vi "Rebuild Addon Settings.vi"(8 "error in (no error)":errorcluster, 11 "Section Ref in":T1 format="%.0x") -> (0 "error out":errorcluster, 3 "Parent Ref out":T1 format="%.0x")   [LabVIEW 2013, in "J1939 Addon System Explorer.lvlib"]
uses:
  J1939 Addon System Explorer.lvlib
  <vilib>/NI Veristand/Custom Device API/Custom Device Item Ref.ctl
  Shared/SubVIs/Constants.vi
  <vilib>/NI Veristand/Custom Device Tools/Custom Device Utility Library/NI VeriStand - Search for Item by Name.vi
  <vilib>/NI Veristand/Custom Device API/Custom Device API.lvlib
  Shared/J1939 Addon Shared.lvlib
  <vilib>/NI Veristand/Custom Device Tools/Custom Device Utility Library/Custom Device Utility Library.lvlib
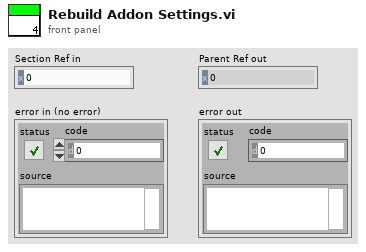
[diagram p1: front panel]
types:
  T1 = typedef "Custom Device API.lvlib/Custom Device Item Ref.ctl" = u64
  T2 = typedef "J1939 Addon Shared.lvlib/XNET Frame Event Properties.ctl" = cluster{"Transmit trigger":enum16{"Channel value change"}, "Enable software cyclic trigger":bool, "Transmit Time":dbl}
  T3 = typedef "J1939 Addon Shared.lvlib/SPN Properties.ctl" = cluster{"Bytes":u32, "ScaleFac":dbl, "ScaleOff":dbl}
  T4 = cluster{"Name":string, "ID":u32, "Frame Transmit Info":T2, "Signal List":cluster{"Name":string, "SPN":T3}[]}[]
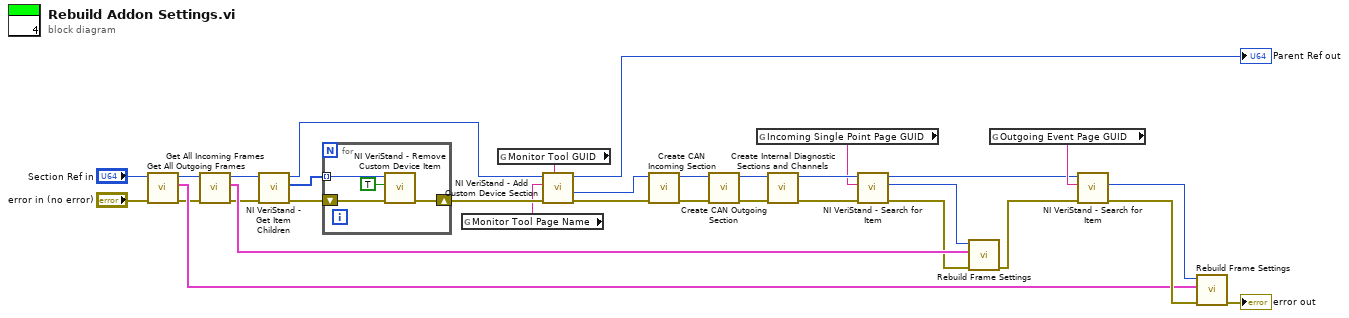
[diagram p0: block diagram]
diagram:
  n1 = call "Get All Outgoing Frames.vi"("error in"="error in (no error)", "Item Ref"="Section Ref in") -> ("error out"=w3:errorcluster, "Frames"=w7:T4, "Item Ref out"=w4:T1)  [unwired: 7 in]
  n2 = call "Get All Incoming Frames.vi"("error in"=w3, "Item Ref"=w4) -> ("error out"=w2:errorcluster, "Frames"=w16:T4, "Item Ref out"=w1:T1)  [unwired: 7 in]
  n3 = call <vilib>:"NI VeriStand - Get Item Children.vi"("error in (no error)"=w2, "Item Ref in"=w1) -> ("error out"=w21:errorcluster, "Child Refs"=w20:T1[], "Item Ref out"=w31:T1)  [unwired: 6 in, 1 out]
  n4 = for {
    tunnel: w20 -> [w36] mode=indexing
    shift-right: [w33] -> w30
    shift-left: w21 -> [w34]
    n5 = call <vilib>:"NI VeriStand - Remove Custom Device Item.vi"("error in (no error)"=w34, "Force Delete (F)"=TRUE, "Item Ref in"=w36) -> ("error out"=w33:errorcluster)  [unwired: 7 in, 1 out]
  }
  n6 = global read "Constants.vi" "Monitor Tool Page Name"() -> (w27:string)
  n7 = global read "Constants.vi" "Monitor Tool GUID"() -> (w26:string)
  n8 = call <vilib>:"NI VeriStand - Add Custom Device Section.vi"("GUID (Default Section)"=w26, "error in (no error)"=w30, "Section Name"=w27, "Parent Ref in"=w31) -> ("error out"=w28:errorcluster, "Section Ptr"=w29:T1, "Parent Ref out"=→"Parent Ref out":T1)  [unwired: 4 in, 1 out]
  n9 = call "Create CAN Incoming Section.vi"("error in (no error)"=w28, "Device Item Ref in"=w29) -> ("error out"=w22:errorcluster, "Device Item Ref Out"=w23:T1)  [unwired: 8 in]
  n10 = call "Create CAN Outgoing Section.vi"("error in (no error)"=w22, "Parent Ref in"=w23) -> ("error out"=w25:errorcluster, "Parent Ref out"=w24:T1)  [unwired: 8 in]
  n11 = global read "Constants.vi" "Incoming Single Point Page GUID"() -> (w17:string)
  n12 = call "Create Internal Diagnostic Sections and Channels.vi"("error in (no error)"=w25, "Device Item Ref in"=w24) -> ("error out"=w19:errorcluster, "Device Item Ref Out"=w18:T1)  [unwired: 8 in]
  n13 = call-poly <vilib>:"NI VeriStand - Search for Item.vi"("error in"=w19, "Item Name"=w17, "Section Ref in"=w18) -> ("error out"=w14:errorcluster, "Item Ref"=w15:T1, "Section Ref out"=w10:T1)  [unwired: 5 in, 1 out]
  n14 = call "Rebuild Frame Settings.vi"("error in (no error)"=w14, "Frames"=w16, "Ref in"=w15) -> ("error out"=w9:errorcluster)  [unwired: 7 in, 1 out]
  n15 = global read "Constants.vi" "Outgoing Event Page GUID"() -> (w11:string)
  n16 = call-poly <vilib>:"NI VeriStand - Search for Item.vi"("error in"=w9, "Item Name"=w11, "Section Ref in"=w10) -> ("error out"=w13:errorcluster, "Item Ref"=w12:T1)  [unwired: 5 in, 2 out]
  n17 = call "Rebuild Frame Settings.vi"("error in (no error)"=w13, "Frames"=w7, "Ref in"=w12) -> ("error out"=→"error out":errorcluster)  [unwired: 7 in, 1 out]
